vi "Read and Write Controls to Library Config File.vi"(7 "Action":T1, 8 "error in":errorcluster, 10 "Control References":refnum<vi>[](array[refnum])) -> (0 "error out":errorcluster)   [LabVIEW 2021]
doc: "Writes the values of an array of controls to a configuration file or reads them back.\n<b>Control References</b> is an array of the references of the controls to be saved.\n\nThe configuration file is named after the VI the first control in the array is in and is saved in the LabVIEW Data folder"
uses:
  RWC_Actions.ctl
  <vilib>/Utility/config.llb/NI_LVConfig.lvlib
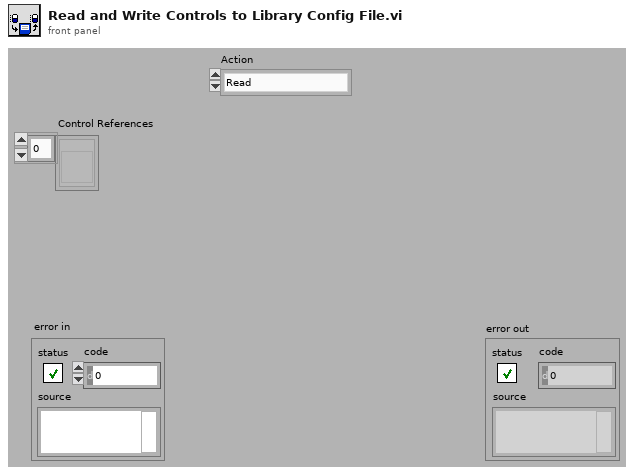
[diagram p1: front panel]
types:
  T1 = typedef "RWC_Actions.ctl" = enum16{"Read", "Write", "Read and Create"}
  T2 = typedef "NI_LVConfig.lvlib/Config Data RefNum.ctl" = refnum<k1>
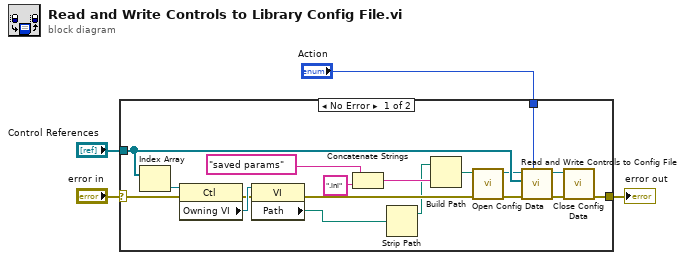
[diagram p0: block diagram]
diagram:
  n1 = case shown="No Error" "error in" {
    selector: "error in" -> [w9 w23]
    tunnel: "Action" -> [w22 _]
    tunnel: "Control References" -> [w21 _]
    tunnel: [w10 w23] -> w1
    frame No Error {
      n2 = Index Array(array=w21) -> (element=w19:refnum<vi>)  [unwired: 1 in]
      n3 = property class="Ctl"(reference=w19, error in=w9) -> (error out=w16:errorcluster, "Owning VI"=w20:refnum<vi>)  [unwired: 1 out]
      n4 = property class="VI"(reference=w20, error in=w16) -> (error out=w15:errorcluster, "Path"=w5:path)  [unwired: 1 out]
      n5 = Concatenate Strings("saved params" ("string"), ".ini" ("string")) -> (w18:string)
      n6 = Strip Path(path=w5) -> (stripped path=w7:path)  [unwired: 1 out]
      n7 = Build Path(base path=w7, name or relative path=w18) -> (appended path=w8:path)
      n8 = call <vilib>:"Open Config Data.vi"("error in (no error)"=w15, "configuration file path"=w8) -> ("error out"=w14:errorcluster, "refnum"=w12:T2)  [unwired: 7 in, 1 out]
      n9 = call "Read and Write Controls to Config File.vi"("Action"=w22, "error in"=w14, "Control References"=w21, "Configuration File Reference In"=w12) -> ("error out"=w11:errorcluster, "Configuration File Reference Out"=w13:T2)  [unwired: 6 in]
      n10 = call <vilib>:"Close Config Data.vi"("error in (no error)"=w11, "refnum"=w13) -> ("error out"=w10:errorcluster)  [unwired: 8 in, 1 out]
    }
    frame Error {
    }
  }
  "error out" <- w1
